vi "总磷总氮控制命令.vi"(8 "Error in":errorcluster caption="Error in (no error)", 11 "参数":T1={"站号"=1, "量程切换"=enum."AUTO", "控制命令"=enum."启动测量", "模式设置"=enum."待机", "测量间隔"=0} {"站号" items=["总磷"=1, "氨氮"=3]}) -> (0 "error out":errorcluster)   [LabVIEW 2016, in "斯坦道总氮V2.lvlib"]
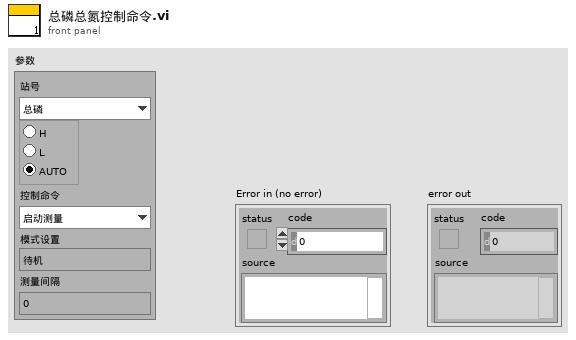
[diagram p1: front panel]
types:
  T1 = cluster{"站号":u16, "量程切换":enum32{"H", "L", "AUTO"}, "控制命令":enum16{"启动测量", "标样核查", "零点核查", "跨度核查", "空白测试", "平行样测试", "加标回收", "空白校准", "标样校准", "初始化（清洗）", "停止测试", "仪器重启", "校时", "模式设置", "测量间隔设置", ""}, "模式设置":enum16{"待机", "连续模式", "周期模式", "定点模式", "受控模式", "手动模式"}, "测量间隔":u16}
  T2 = enum16{"启动测量", "标样核查", "零点核查", "跨度核查", "空白测试", "平行样测试", "加标回收", "空白校准", "标样校准", "初始化（清洗）", "停止测试", "仪器重启", "校时", "模式设置", "测量间隔设置", ""}
  T3 = enum16{"待机", "连续模式", "周期模式", "定点模式", "受控模式", "手动模式"}
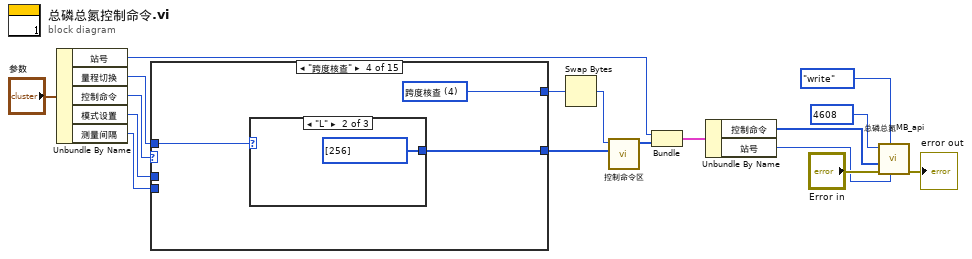
[diagram p0: block diagram]
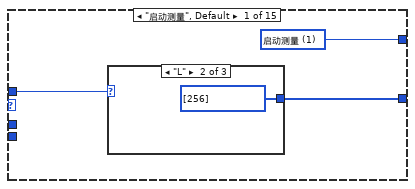
[diagram p2: hidden frame]
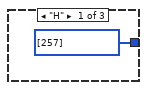
[diagram p3: hidden frame]
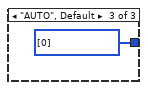
[diagram p4: hidden frame]
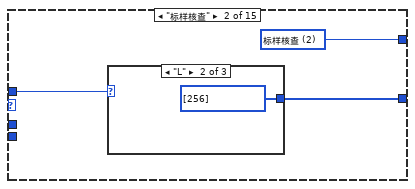
[diagram p5: hidden frame]
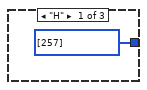
[diagram p6: hidden frame]
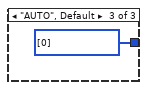
[diagram p7: hidden frame]
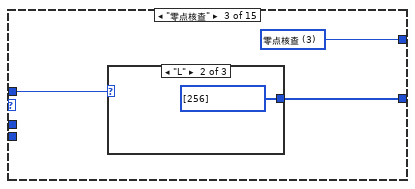
[diagram p8: hidden frame]
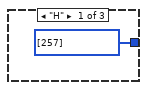
[diagram p9: hidden frame]
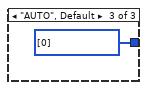
[diagram p10: hidden frame]
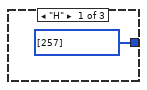
[diagram p11: hidden frame]
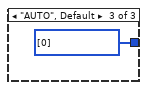
[diagram p12: hidden frame]
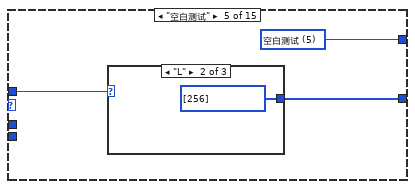
[diagram p13: hidden frame]
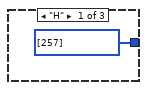
[diagram p14: hidden frame]
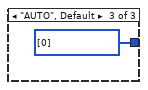
[diagram p15: hidden frame]
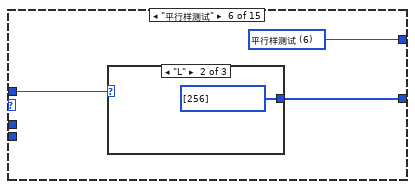
[diagram p16: hidden frame]
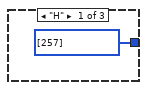
[diagram p17: hidden frame]
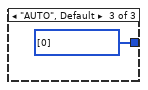
[diagram p18: hidden frame]
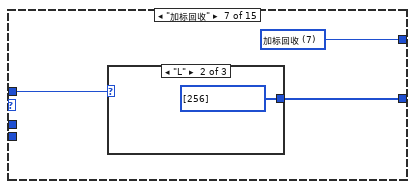
[diagram p19: hidden frame]
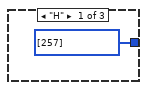
[diagram p20: hidden frame]
diagram:
  n1 = Unbundle By Name("参数") -> ("站号"=w12:u16, "量程切换"=w11:enum32{"H", "L", "AUTO"}, "控制命令"=w10:T2, "模式设置"=w8:T3, "测量间隔"=w9:u16)
  n2 = case shown="\"跨度核查\"" w10 {
    tunnel: [w18 w24 w30 w36 w42 w48 w54 w60 w66 i32[] [] i32[] [] i32[] [] w78 w84 w94] -> w3
    tunnel: w11 -> [w20 w26 w32 w38 w44 w50 w56 w62 w68 _ _ _ _ _ _]
    tunnel: [w19 w25 w31 w37 w43 w49 w55 w61 w67 w72 w74 w76 w79 w86 w96] -> w2
    tunnel: w9 -> [_ _ _ _ _ _ _ _ _ _ _ _ _ _ w93]
    tunnel: w8 -> [_ _ _ _ _ _ _ _ _ _ _ _ _ w83 _]
    frame "启动测量", Default {
      w19 = u16 1 items=["启动测量"=1, "标样核查"=2, "零点核查"=3, "跨度核查"=4, "空白测试"=5, "平行样测试"=6, "加标回收"=7, "空白校准"=8, "标样校准"=9, "初始化（清洗）"=10, "停止测试"=11, "仪器重启"=12, "校时"=13, "模式设置"=14, "测量间隔设置"=15] ("控制命令")
      n3 = case shown="\"L\"" w20 {
        tunnel: [i32[] [257] i32[] [256] i32[] [0]] -> w18
        frame "H" {
        }
        frame "L" {
        }
        frame "AUTO", Default {
        }
      }
    }
    frame "标样核查" {
      w25 = u16 2 items=["启动测量"=1, "标样核查"=2, "零点核查"=3, "跨度核查"=4, "空白测试"=5, "平行样测试"=6, "加标回收"=7, "空白校准"=8, "标样校准"=9, "初始化（清洗）"=10, "停止测试"=11, "仪器重启"=12, "校时"=13, "模式设置"=14, "测量间隔设置"=15] ("控制命令")
      n4 = case shown="\"L\"" w26 {
        tunnel: [i32[] [257] i32[] [256] i32[] [0]] -> w24
        frame "H" {
        }
        frame "L" {
        }
        frame "AUTO", Default {
        }
      }
    }
    frame "零点核查" {
      w31 = u16 3 items=["启动测量"=1, "标样核查"=2, "零点核查"=3, "跨度核查"=4, "空白测试"=5, "平行样测试"=6, "加标回收"=7, "空白校准"=8, "标样校准"=9, "初始化（清洗）"=10, "停止测试"=11, "仪器重启"=12, "校时"=13, "模式设置"=14, "测量间隔设置"=15] ("控制命令")
      n5 = case shown="\"L\"" w32 {
        tunnel: [i32[] [257] i32[] [256] i32[] [0]] -> w30
        frame "H" {
        }
        frame "L" {
        }
        frame "AUTO", Default {
        }
      }
    }
    frame "跨度核查" {
      w37 = u16 4 items=["启动测量"=1, "标样核查"=2, "零点核查"=3, "跨度核查"=4, "空白测试"=5, "平行样测试"=6, "加标回收"=7, "空白校准"=8, "标样校准"=9, "初始化（清洗）"=10, "停止测试"=11, "仪器重启"=12, "校时"=13, "模式设置"=14, "测量间隔设置"=15] ("控制命令")
      n6 = case shown="\"L\"" w38 {
        tunnel: [i32[] [257] i32[] [256] i32[] [0]] -> w36
        frame "H" {
        }
        frame "L" {
        }
        frame "AUTO", Default {
        }
      }
    }
    frame "空白测试" {
      w43 = u16 5 items=["启动测量"=1, "标样核查"=2, "零点核查"=3, "跨度核查"=4, "空白测试"=5, "平行样测试"=6, "加标回收"=7, "空白校准"=8, "标样校准"=9, "初始化（清洗）"=10, "停止测试"=11, "仪器重启"=12, "校时"=13, "模式设置"=14, "测量间隔设置"=15] ("控制命令")
      n7 = case shown="\"L\"" w44 {
        tunnel: [i32[] [257] i32[] [256] i32[] [0]] -> w42
        frame "H" {
        }
        frame "L" {
        }
        frame "AUTO", Default {
        }
      }
    }
    frame "平行样测试" {
      w49 = u16 6 items=["启动测量"=1, "标样核查"=2, "零点核查"=3, "跨度核查"=4, "空白测试"=5, "平行样测试"=6, "加标回收"=7, "空白校准"=8, "标样校准"=9, "初始化（清洗）"=10, "停止测试"=11, "仪器重启"=12, "校时"=13, "模式设置"=14, "测量间隔设置"=15] ("控制命令")
      n8 = case shown="\"L\"" w50 {
        tunnel: [i32[] [257] i32[] [256] i32[] [0]] -> w48
        frame "H" {
        }
        frame "L" {
        }
        frame "AUTO", Default {
        }
      }
    }
    frame "加标回收" {
      w55 = u16 7 items=["启动测量"=1, "标样核查"=2, "零点核查"=3, "跨度核查"=4, "空白测试"=5, "平行样测试"=6, "加标回收"=7, "空白校准"=8, "标样校准"=9, "初始化（清洗）"=10, "停止测试"=11, "仪器重启"=12, "校时"=13, "模式设置"=14, "测量间隔设置"=15] ("控制命令")
      n9 = case shown="\"L\"" w56 {
        tunnel: [i32[] [257] i32[] [256] i32[] [0]] -> w54
        frame "H" {
        }
        frame "L" {
        }
        frame "AUTO", Default {
        }
      }
    }
    frame "空白校准" {
      w61 = u16 8 items=["启动测量"=1, "标样核查"=2, "零点核查"=3, "跨度核查"=4, "空白测试"=5, "平行样测试"=6, "加标回收"=7, "空白校准"=8, "标样校准"=9, "初始化（清洗）"=10, "停止测试"=11, "仪器重启"=12, "校时"=13, "模式设置"=14, "测量间隔设置"=15] ("控制命令")
      n10 = case shown="\"L\"" w62 {
        tunnel: [i32[] [257] i32[] [256] i32[] [0]] -> w60
        frame "H" {
        }
        frame "L" {
        }
        frame "AUTO", Default {
        }
      }
    }
    frame "标样校准" {
      w67 = u16 9 items=["启动测量"=1, "标样核查"=2, "零点核查"=3, "跨度核查"=4, "空白测试"=5, "平行样测试"=6, "加标回收"=7, "空白校准"=8, "标样校准"=9, "初始化（清洗）"=10, "停止测试"=11, "仪器重启"=12, "校时"=13, "模式设置"=14, "测量间隔设置"=15] ("控制命令")
      n11 = case shown="\"L\"" w68 {
        tunnel: [i32[] [257] i32[] [256] i32[] [0]] -> w66
        frame "H" {
        }
        frame "L" {
        }
        frame "AUTO", Default {
        }
      }
    }
    frame "初始化（清洗）" {
      w72 = u16 10 items=["启动测量"=1, "标样核查"=2, "零点核查"=3, "跨度核查"=4, "空白测试"=5, "平行样测试"=6, "加标回收"=7, "空白校准"=8, "标样校准"=9, "初始化（清洗）"=10, "停止测试"=11, "仪器重启"=12, "校时"=13, "模式设置"=14, "测量间隔设置"=15] ("控制命令")
    }
    frame "停止测试" {
      w74 = u16 11 items=["启动测量"=1, "标样核查"=2, "零点核查"=3, "跨度核查"=4, "空白测试"=5, "平行样测试"=6, "加标回收"=7, "空白校准"=8, "标样校准"=9, "初始化（清洗）"=10, "停止测试"=11, "仪器重启"=12, "校时"=13, "模式设置"=14, "测量间隔设置"=15] ("控制命令")
    }
    frame "仪器重启" {
      w76 = u16 12 items=["启动测量"=1, "标样核查"=2, "零点核查"=3, "跨度核查"=4, "空白测试"=5, "平行样测试"=6, "加标回收"=7, "空白校准"=8, "标样校准"=9, "初始化（清洗）"=10, "停止测试"=11, "仪器重启"=12, "校时"=13, "模式设置"=14, "测量间隔设置"=15] ("控制命令")
    }
    frame "校时" {
      w79 = u16 13 items=["启动测量"=1, "标样核查"=2, "零点核查"=3, "跨度核查"=4, "空白测试"=5, "平行样测试"=6, "加标回收"=7, "空白校准"=8, "标样校准"=9, "初始化（清洗）"=10, "停止测试"=11, "仪器重启"=12, "校时"=13, "模式设置"=14, "测量间隔设置"=15] ("控制命令")
      n12 = Get Date/Time In Seconds() -> (seconds since 1Jan1904=w82:timestamp)
      n13 = Insert Into Array(array=timestamp[] [] ("数组"), new element=w82) -> (w80:timestamp[])  [unwired: 1 in]
      n14 = call "DateToHex.vi"("DATE"=w80) -> ("数组"=w78:u16[])  [unwired: 10 in]
    }
    frame "模式设置" {
      w86 = u16 14 items=["启动测量"=1, "标样核查"=2, "零点核查"=3, "跨度核查"=4, "空白测试"=5, "平行样测试"=6, "加标回收"=7, "空白校准"=8, "标样校准"=9, "初始化（清洗）"=10, "停止测试"=11, "仪器重启"=12, "校时"=13, "模式设置"=14, "测量间隔设置"=15] ("控制命令")
      n15 = case shown="\"手动模式\"" w83 {
        tunnel: [i32[] [0] i32[] [1] i32[] [2] i32[] [3] i32[] [4] i32[] [5]] -> w85
        frame "待机", Default {
        }
        frame "连续模式" {
        }
        frame "周期模式" {
        }
        frame "定点模式" {
        }
        frame "受控模式" {
        }
        frame "手动模式" {
        }
      }
      n16 = call "HexToWord.vi"("数组"=w85) -> ("WORD"=w84:u16[])  [unwired: 10 in]
    }
    frame "测量间隔设置" {
      w96 = u16 15 items=["启动测量"=1, "标样核查"=2, "零点核查"=3, "跨度核查"=4, "空白测试"=5, "平行样测试"=6, "加标回收"=7, "空白校准"=8, "标样校准"=9, "初始化（清洗）"=10, "停止测试"=11, "仪器重启"=12, "校时"=13, "模式设置"=14, "测量间隔设置"=15] ("控制命令")
      n17 = Replace Array Subset(array=i32[] [0], new element=w93) -> (w95:i32[])  [unwired: 1 in]
      n18 = call "HexToWord.vi"("数组"=w95) -> ("WORD"=w94:u16[])  [unwired: 10 in]
    }
  }
  n19 = Swap Bytes(anything=w2) -> (byte swapped=w1:u16)
  n20 = call "控制命令区.vi"("控制命令参数"=w3, "控制命令"=w1) -> ("控制命令"=w4:u16[])  [unwired: 9 in]
  n21 = Bundle("站号"=w12, "控制命令"=w4) -> (w7:cluster{"站号":u16, "控制命令":u16[]})  [unwired: 1 in]
  n22 = Unbundle By Name(w7) -> ("控制命令"=w6:u16[], "站号"=w5:u16)
  n23 = call "总磷总氮MB_api.vi"("Slave ID"=w5, "STEP"=enum16{"open", "read", "write", "close"}."write", "Error in"="Error in", "values"=w6, "starting address"=u16 4608) -> ("error out"=→"error out":errorcluster)  [unwired: 4 in, 2 out]
